vi "Read U64 Direct Dispatch.vi"(8 "error in (no error)":errorcluster, 9 "Timeout (ms)":i32, 11 "CIFTag in":refnum<class "CIFChannels.lvclass">) -> (0 "error out":errorcluster, 1 "timed out?":bool, 2 "Data":u64, 3 "CIFTag out":refnum<class "CIF_NIChn_U64.lvclass">)   [LabVIEW 2021, in "CIF_NIChn_U64.lvclass"]
uses:
  CIF_NIChn_U64.lvclass
  CIF_NIChn_U64.lvclass/CIF_NIChn_U64.ctl
  CIFChannels/Typedef/Direction.ctl
  CIFChannels/CIFChannels.lvclass
  CIFChannels/Typedef/Channel State.ctl
  NIChn/CIF_NIChn.lvclass
  cbead010-ab61-49ec-ac6c-083511305d37.vi
  D:/dev/Packages/Channel_Manager/src/CIF_NIChn/NIChn/CIF_NIChn.lvclass
  D:/dev/Packages/Channel_Manager/src/CIFChannels/CIFChannels.lvclass
  D:/dev/Packages/Channel_Manager/src/CIF_NIChn/U64/CIF_NIChn_U64.lvclass
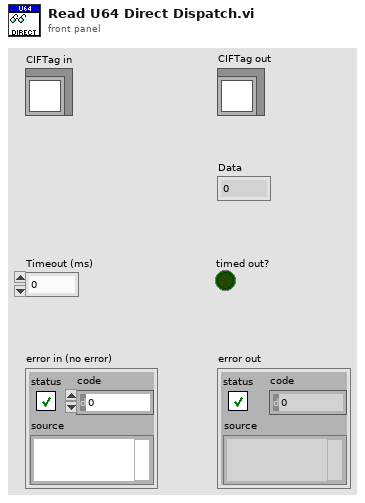
[diagram p1: front panel]
types:
  T1 = typedef "CIFChannels.lvclass/Channel State.ctl" = enum16{"Creating", "Disconnected", "Connecting", "Connected", "Destroyed"}
  T2 = typedef "CIFChannels.lvclass/Direction.ctl" = enum16{"Publisher", "Subscriber"}
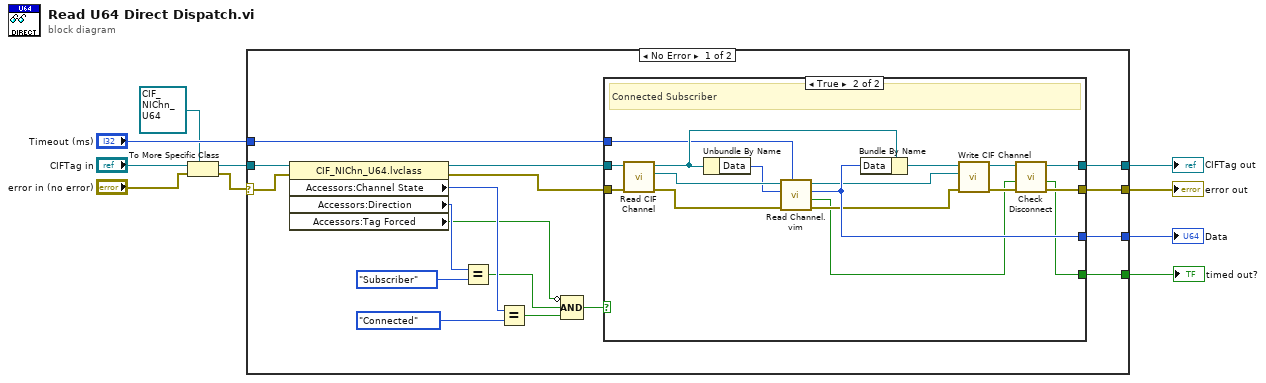
[diagram p0: block diagram]
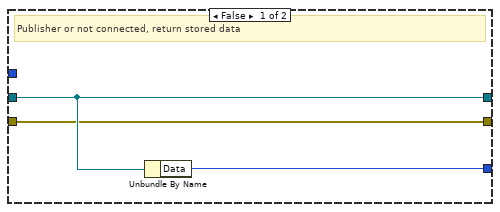
[diagram p2: hidden frame]
diagram:
  n1 = To More Specific Class(target class=refnum<class "CIF_NIChn_U64.lvclass"> refnum ("CIFTag in"), reference="CIFTag in", error in="error in (no error)") -> (specific class reference=w3:refnum<class "CIF_NIChn_U64.lvclass">, error out=w1:errorcluster)
  n2 = case shown="No Error" w1 {
    selector: w1 -> [w24 w49]
    tunnel: [w13 w49] -> w10
    tunnel: [w14 w48] -> w9
    tunnel: w3 -> [w25 w48]
    tunnel: [w27 _] -> w8
    tunnel: [w26 _] -> w7
    tunnel: "Timeout (ms)" -> [w12 _]
    frame No Error {
      n3 = property class="CIF_NIChn_U64.lvclass"(reference=w25, error in=w24) -> (reference out=w23:refnum<class "CIF_NIChn_U64.lvclass">, error out=w22:errorcluster, "Accessors:Channel State"=w19:T1, "Accessors:Direction"=w21:T2, "Accessors:Tag Forced"=w11:bool)
      n4 = Equal?(x=w21, y=Direction."Subscriber") -> (x = y?=w15:bool)
      n5 = Equal?(x=w19, y=Channel_State."Connected") -> (x = y?=w17:bool)
      n6 = Compound Arithmetic op=AND(invert w11, w15, w17) -> (w16:bool)
      n7 = case shown="True" w16 {
        tunnel: [_ w33] -> w27
        tunnel: [w30 w40] -> w26
        tunnel: w22 -> [w28 w46]
        tunnel: w23 -> [w29 w47]
        tunnel: [w29 w45] -> w14
        tunnel: [w28 w44] -> w13
        tunnel: w12 -> [_ w32]
        frame False {
          # "Publisher or not connected, return stored data"
          n8 = Unbundle By Name(w29) -> ("Data"=w30:u64)
        }
        frame True {
          # "Connected Subscriber"
          n9 = call "Read CIF Channel.vi"("error in (no error)"=w46, "CIFTag in"=w47) -> ("error out"=w41:errorcluster, "CIF Channel"=w42:refnum<k21>, "CIFTag out"=w43:refnum<class "CIF_NIChn_U64.lvclass">)  [unwired: 7 in]
          n10 = Unbundle By Name(w43) -> ("Data"=w31:u64)
          n11 = call "Read Channel.vim"("Timeout (ms)"=w32, "error in"=w41, "Data in"=w31, "CIF Channel in"=w42) -> ("error out"=w38:errorcluster, "Timed out?"=w34:bool, "Data out"=w40:u64, "CIF Channel out"=w37:refnum<k21>)  [unwired: 4 in]
          n12 = Bundle By Name(cluster=w43, "Data"=w40) -> (w39:refnum<class "CIF_NIChn_U64.lvclass">)
          n13 = call "Write CIF Channel.vi"("error in (no error)"=w38, "CIF Channel"=w37, "CIFTag in"=w39) -> ("error out"=w35:errorcluster, "CIFTag out"=w36:refnum<class "CIF_NIChn_U64.lvclass">)  [unwired: 7 in]
          n14 = call "Check Disconnect.vi"("error in (no error)"=w35, "timeout in"=w34, "CIFTag in"=w36) -> ("error out"=w44:errorcluster, "timeout out"=w33:bool, "CIFTag out"=w45:refnum<class "CIF_NIChn_U64.lvclass">)  [unwired: 5 in, 1 out]
        }
      }
    }
    frame Error {
    }
  }
  "error out" <- w10
  "CIFTag out" <- w9
  "timed out?" <- w8
  "Data" <- w7
